vi "EXP6 (Access given & denied).vi"() -> ()   [LabVIEW 2024]
panel:
  out "Access denied":bool
  out "Access given":bool
  out "Username":string
  in  "Table Control":string[][](table)
  in  "Password":string
  in  "Name":string
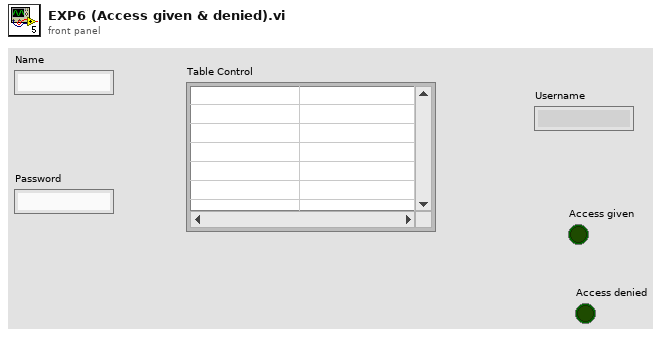
[diagram p1: front panel]
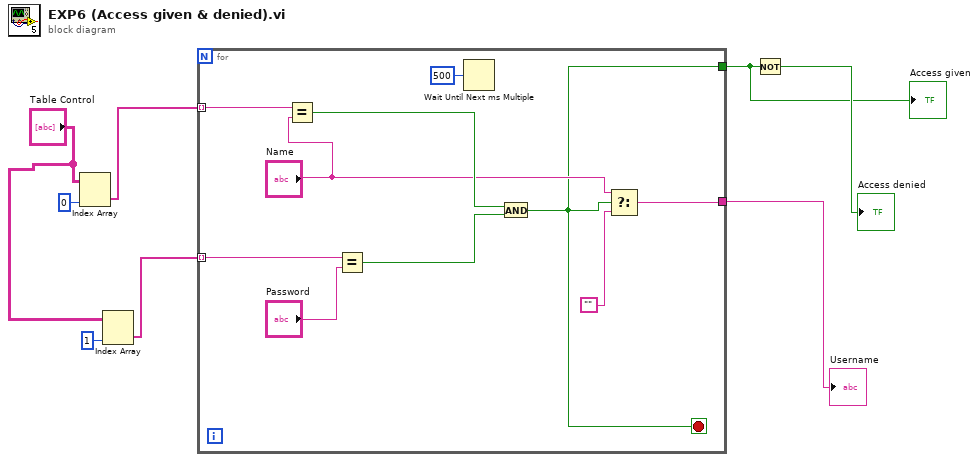
[diagram p0: block diagram]
diagram:
  n1 = Index Array(array="Table Control", index (col)=0 ("disabled index (col)")) -> (element=w5:string[])  [unwired: 1 in]
  n2 = Index Array(array="Table Control", index (col)=1 ("disabled index (col)")) -> (element=w4:string[])  [unwired: 1 in]
  n3 = for {
    tunnel: w5 -> [w18] mode=indexing
    tunnel: w4 -> [w17] mode=indexing
    tunnel: [w10] -> w1
    tunnel: [w9] -> w3
    stop <- w10 stop-if-true
    n4 = Equal?(x=w18, y="Name") -> (x = y?=w15:bool)
    n5 = Equal?(x=w17, y="Password") -> (x = y?=w14:bool)
    n6 = Wait Until Next ms Multiple(millisecond multiple=u32 500) -> ()  [unwired: 1 out]
    n7 = And(x=w15, y=w14) -> (x .and. y?=w10:bool)
    n8 = Select(t="Name", s=w10, f="") -> (s? t:f=w9:string)
  }
  "Username" <- w3
  "Access given" <- w1
  n9 = Not(x=w1) -> (.not. x?=→"Access denied":bool)
